vi "Demo v7_QL.vi"() -> ()   [LabVIEW 2013]
panel:
  out "Biggest score":i32
  in  "Reset score":bool
  in  "Reset x":bool
  out "Biggest x":i32
  out "Bird height":i32
  in  "ms to wait":u32=1000
  out "0, 1":i16[](graph)
  out "Out of bound":bool
  out "Hit tube":bool
  out "Unrolled state":i32
  out "Brid x":i32
  out "Iteration":i32
  out "Q":dbl[][](array[numeric])
  in  "Slow":bool=TRUE
  in  "stop":bool
  out "JUMP?":bool
  out "SCORE":i32
  out "FAIL!":bool
  in  "a":dbl=-0.3
  in  "Jump speed":dbl=3.0
  out "Picture":i32[][](graph)
  # "JUMP"
  # "FALL"
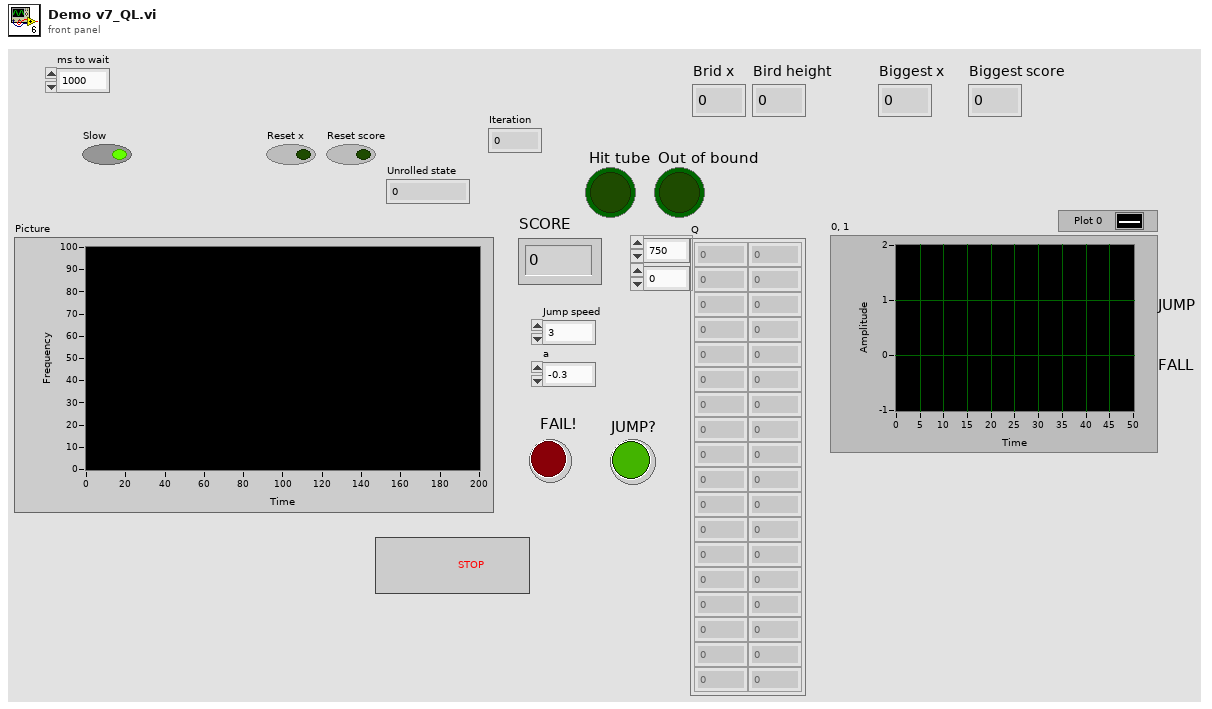
[diagram p1: front panel]
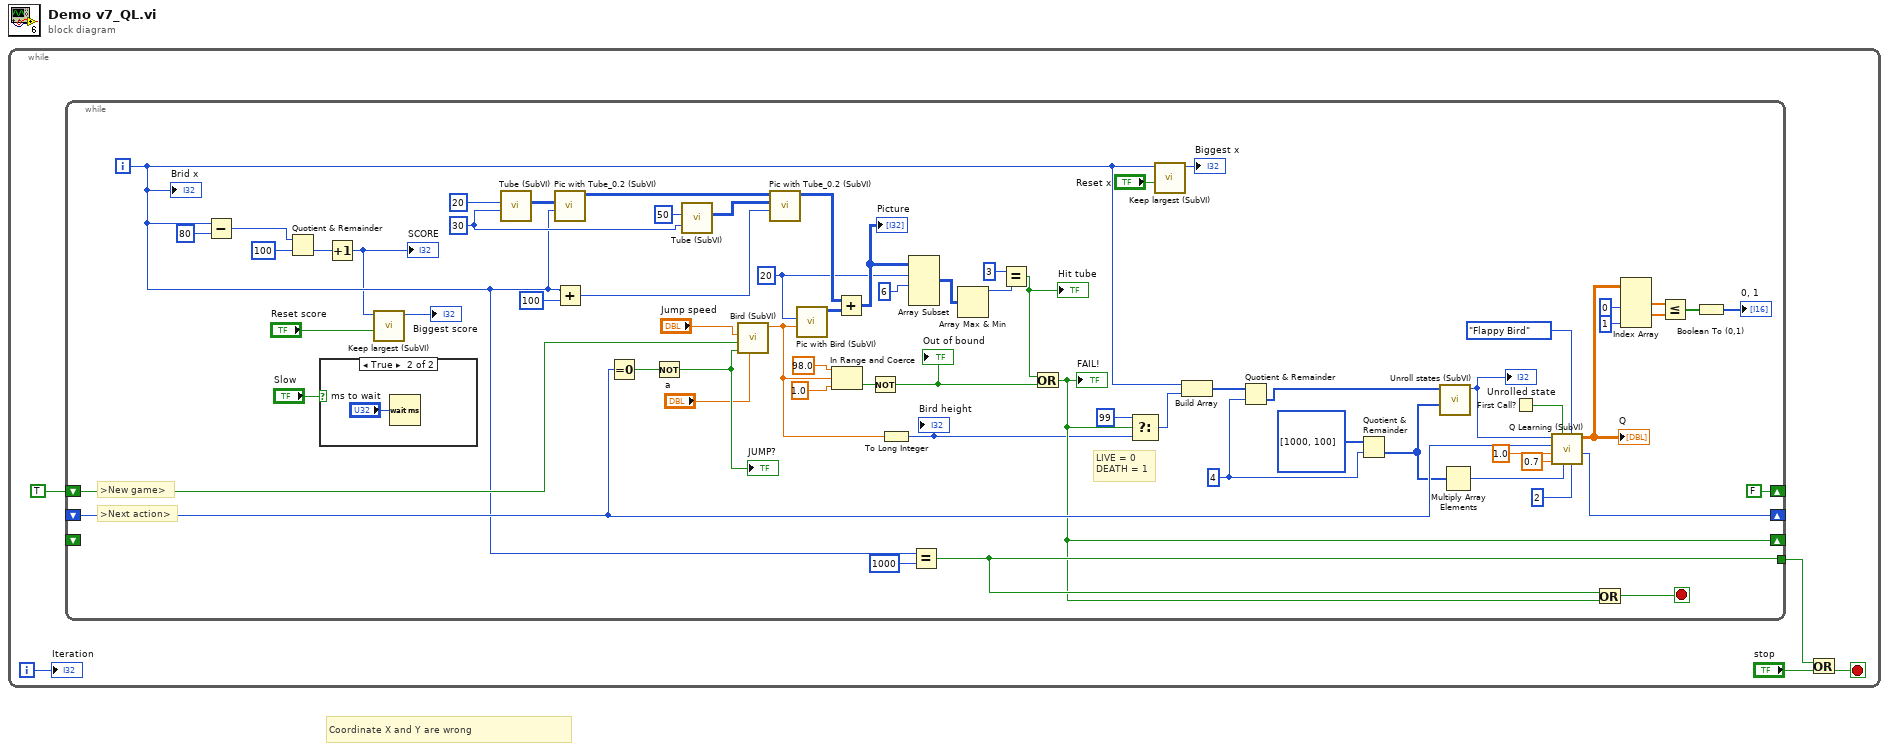
[diagram p0: block diagram]
diagram:
  # "Coordinate X and Y are wrong"
  n1 = while {
    i -> [w4]
    stop <- w3 stop-if-true
    n2 = while {
      shift-right: [w29] -> _
      shift-left: _ -> [_]
      tunnel: [w44] -> w2
      shift-right: [FALSE] -> _
      shift-left: TRUE -> [w34]
      shift-right: [w32] -> _
      shift-left: _ -> [w31]
      i -> [w26]
      stop <- w45 stop-if-true
      w9 = 4 ("s? t:f")
      w20 = 20 ("X position")
      w68 = 30 ("Gap height (30)")
      # ">New game>"
      # ">Next action>"
      # "LIVE = 0\nDEATH = 1"
      n3 = Subtract(x=w26, y=80) -> (x-y=w60:i32)
      n4 = Quotient & Remainder(x=w60, y=100) -> (floor(x/y)=w16:i32)  [unwired: 1 out]
      n5 = case shown="True" "Slow" {
        frame False {
        }
        frame True {
          n6 = Wait (ms)(milliseconds to wait="ms to wait") -> ()  [unwired: 1 out]
        }
      }
      n7 = Increment(x=w16) -> (x+1=w14:i32)
      "SCORE" <- w14
      n8 = call "Keep largest (SubVI).vi"("Reset"="Reset score", "Input"=w14) -> ("Biggest"=→"Biggest score":i32)  [unwired: 9 in]
      n9 = call "Tube (SubVI).vi"("Gap height (30)"=w68, "Gap low y"=20) -> ("Tube"=w70:i32[][])  [unwired: 9 in]
      n10 = call "Pic with Tube_0.2 (SubVI).vi"("Tube x"=w26, "Tube"=w70) -> ("Picture"=w69:i32[][])  [unwired: 9 in]
      n11 = Add(x=w26, y=100) -> (x+y=w48:i32)
      n12 = Equal To 0?(x=w31) -> (x = 0?=w56:bool)
      n13 = Not(x=w56) -> (.not. x?=w55:bool)
      "JUMP?" <- w55
      n14 = call "Tube (SubVI).vi"("Gap height (30)"=w68, "Gap low y"=50) -> ("Tube"=w36:i32[][])  [unwired: 9 in]
      n15 = call "Bird (SubVI).vi"("a"="a", "Jump"=w55, "Reset"=w34, "Jump speed"="Jump speed") -> ("Position"=w30:dbl)  [unwired: 7 in]
      n16 = call "Pic with Tube_0.2 (SubVI).vi"("Tube x"=w48, "Tube"=w36, "Picture in"=w69) -> ("Picture"=w50:i32[][])  [unwired: 8 in]
      n17 = call "Pic with Bird (SubVI).vi"("Bird Position"=w30, "X position"=w20) -> ("Picture"=w72:i32[][])  [unwired: 9 in]
      n18 = In Range and Coerce(upper limit=98.0, x=w30, lower limit=1.0) -> (In Range?=w65:bool)  [unwired: 1 out]
      n19 = Add(x=w50, y=w72) -> (x+y=w21:i32[][])
      "Picture" <- w21
      n20 = Not(x=w65) -> (.not. x?=w63:bool)
      "Out of bound" <- w63
      n21 = To Long Integer(number=w30) -> (32bit integer=w6:i32)
      "Bird height" <- w6
      n22 = Array Subset(array=w21, index (row)=w20, length (row)=6 ("length")) -> (w18:i32[][])  [unwired: 2 in]
      n23 = Equal?(x=w26, y=1000) -> (x = y?=w44:bool)
      n24 = Array Max & Min(array=w18) -> (max value=w17:i32)  [unwired: 3 out]
      n25 = Equal?(x=3 ("y"), y=w17) -> (x = y?=w51:bool)
      "Hit tube" <- w51
      n26 = Or(x=w51, y=w63) -> (x .or. y?=w29:bool)
      "FAIL!" <- w29
      n27 = Select(t=99, s=w29, f=w6) -> (s? t:f=w28:i32)
      n28 = call "Keep largest (SubVI).vi"("Reset"="Reset x", "Input"=w26) -> ("Biggest"=→"Biggest x":i32)  [unwired: 9 in]
      n29 = Build Array(w26, w28) -> (w57:i32[])
      n30 = Quotient & Remainder(x=w57, y=w9) -> (floor(x/y)=w11:i32[])  [unwired: 1 out]
      n31 = Quotient & Remainder(x=i32[] [1000, 100] ("# each state"), y=w9) -> (floor(x/y)=w8:i32[])  [unwired: 1 out]
      n32 = call "Unroll states (SubVI).vi"("size of each state"=w8, "State array"=w11) -> ("Unrolled state"=w24:i32)  [unwired: 9 in]
      "Unrolled state" <- w24
      n33 = Multiply Array Elements(1:w8) -> (0:w7:i32)
      n34 = First Call?() -> (First Call?: T/F=w12:bool)
      n35 = call "Q Learning (SubVI).vi"("# action"=2, "Mode"=enum16{"Algorithm test", "Flappy Bird"}."Flappy Bird", "# state"=w7, "Reset"=w12, "alpha"=0.7, "Gamma"=1.0, "Action"=w31, "State"=w24) -> ("Next Action"=w32:i32, "Q"=w43:dbl[][])  [unwired: 2 in]
      "Q" <- w43
      n36 = Or(x=w44, y=w29) -> (x .or. y?=w45:bool)
      n37 = Index Array(array=w43, index (col) #1=0 ("disabled index (col)"), index (col) #2=1 ("index (col)")) -> (element #1=w40:dbl[], element #2=w39:dbl[])  [unwired: 2 in]
      n38 = Less Or Equal?(x=w40, y=w39) -> (x <= y?=w38:bool[])
      n39 = Boolean To (0,1)(Boolean=w38) -> (0, 1=→"0, 1":i16[])
      "Brid x" <- w26
    }
    n40 = Or(x=w2, y="stop") -> (x .or. y?=w3:bool)
    "Iteration" <- w4
  }
